vi "Load Single Level.vi"(8 "error in (no error)":errorcluster, 10 "Tag":string, 11 "TreeDirectory in":refnum<class "TreeDirectoryExt.lvclass">) -> (0 "error out":errorcluster, 3 "Tree (dup)":refnum<class "TreeDirectoryExt.lvclass">)   [LabVIEW 2026, in "TreeDirectoryExt.lvclass"]
uses:
  TreeDirectoryExt.lvclass
  C:/Program Files/National Instruments/LabVIEW 2026/vi.lib/QSI/QControls/QControl Classes/TreeControl/TreeControl.lvclass
  <vilib>/QSI/QControls/QControl Classes/TreeControl/Add Item Info Cluster.ctl
  TreeDirectoryExt.lvclass/TreeDirectoryExt.ctl
  <vilib>/QSI/QControls/QControl Classes/TreeControl/Tree Action Enum.ctl
  <vilib>/QSI/QControls/QControl Classes/TreeControl/TreeControl.lvclass
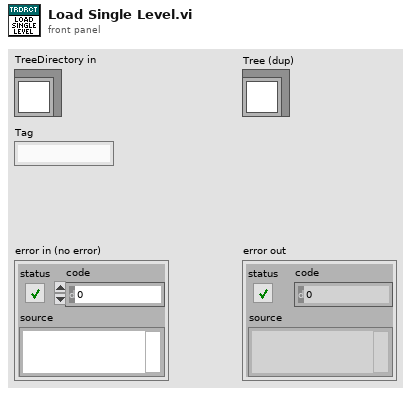
[diagram p1: front panel]
types:
  T1 = typedef "TreeControl.lvclass/Add Item Info Cluster.ctl" = cluster{"Parent Tag (\"\")":string, "Child Position (-1=End)":i32, "Left Cell String (\"\" = Same as Child Tag)":string, "Child Text[]":string[], "Child Tag":string, "Child Only? (F)":bool}
  T2 = typedef "TreeControl.lvclass/Tree Action Enum.ctl" = enum16{"Open All", "Close All", "Open Item", "Close Item"}
  T3 = typedef "imagedata.ctl" = cluster{"image type":i32, "image depth":i32, "image":u8[], "mask":u8[], "colors":u32[], "Rectangle":cluster{"left":i16, "top":i16, "right":i16, "bottom":i16}}
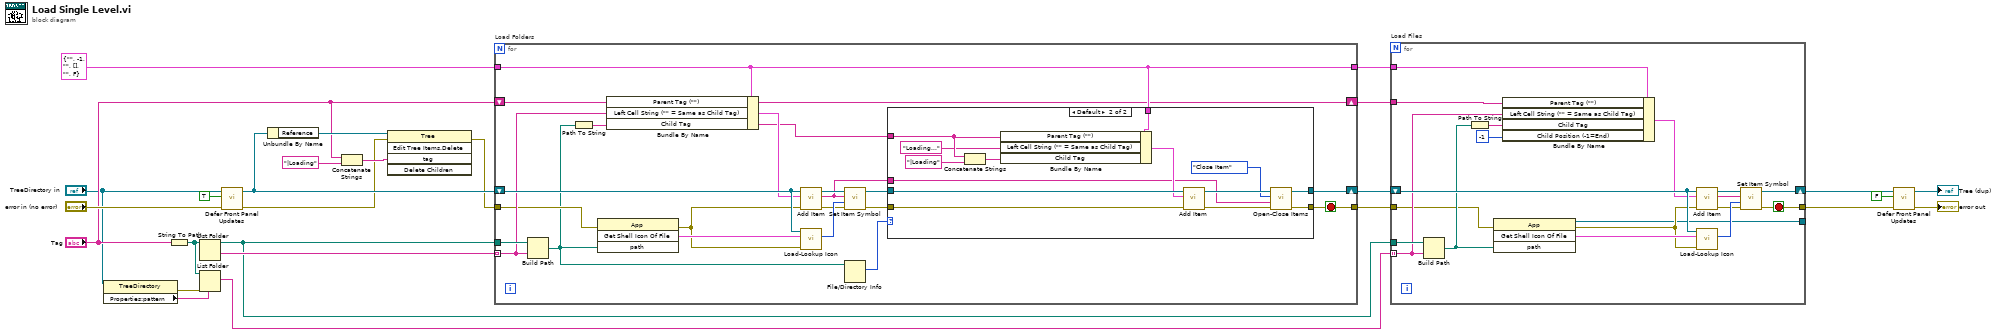
[diagram p0: block diagram]
diagram:
  n1 = property class="TreeDirectory"(reference="TreeDirectory in") -> (error out=w1:errorcluster, "Properties:pattern"=w2:string)  [unwired: 1 in, 1 out]
  n2 = String To Path(string="Tag") -> (path=w5:path)
  n3 = List Folder(path=w5) -> (path out=w21:path, folder names=w26:string[])  [unwired: 3 in, 2 out]
  n4 = List Folder(path=w5, pattern=w2, error in=w1) -> (filenames=w4:string[])  [unwired: 1 in, 3 out]
  n5 = call <vilib>:"Defer Front Panel Updates.vi"("error in (no error)"="error in (no error)", "Defer Panel Updates (F)"=TRUE, "Tree in"="TreeDirectory in") -> ("error out"=w13:errorcluster, "Tree (dup)"=w17:refnum<class "TreeDirectoryExt.lvclass">)  [unwired: 7 in]
  n6 = Unbundle By Name(w17) -> ("Reference"=w16:refnum<vi>)
  n7 = Concatenate Strings("Tag", "|Loading" ("string")) -> (w14:string)
  n8 = invoke class="Tree" method="Edit Tree Items.Delete"(reference=w16, error in=w13, "tag"=w14) -> (error out=w12:errorcluster)  [unwired: 2 in, 4 out]
  n9 = for "Load Folders" {
    tunnel: w26 -> [w42] mode=indexing
    shift-right: [w34] -> w25
    shift-left: w17 -> [w44]
    tunnel: w21 -> [w46]
    tunnel: T1 {"Parent Tag (\"\")"="", "Child Position (-1=End)"=-1, "Left Cell String (\"\" = Same as Child Tag)"="", "Child Text[]"=[], "Child Tag"="", "Child Only? (F)"=FALSE} ("ItemInfo") -> [w36]
    tunnel: [w36] -> w23
    tunnel: [w33] -> w7
    tunnel: w12 -> [w32]
    shift-right: [w29] -> w22
    shift-left: "Tag" -> [w29]
    stop <- w33 stop-if-true
    n10 = Build Path(base path=w46, name or relative path=w42) -> (appended path=w28:path)
    n11 = Path To String(path=w28) -> (string=w40:string)
    n12 = invoke class="App" method="Get Shell Icon Of File"(error in=w32, "path"=w28) -> (error out=w30:errorcluster, "GetShellIconOfFile"=w31:T3)  [unwired: 2 in, 2 out]
    n13 = Bundle By Name(cluster=w36, "Parent Tag (\"\")"=w29, "Left Cell String (\"\" = Same as Child Tag)"=w42, "Child Tag"=w40) -> (w41:T1)
    n14 = call-dynamic "Add Item.vi"("error in (no error)"=w30, "ItemInfo"=w41, "Tree in"=w44) -> ("error out"=w37:errorcluster, "Add Item Tag"=w35:string, "Tree (dup)"=w43:refnum<class "TreeDirectoryExt.lvclass">)  [unwired: 6 in]
    n15 = call "Load-Lookup Icon.vi"("error in (no error)"=w30, "Shell Icon"=w31, "TreeDirectory in"=w44) -> ("Icon Index"=w45:i32)  [unwired: 6 in, 2 out]
    n16 = call <vilib>:"Set Item Symbol.vi"("error in (no error)"=w37, "Symbol Index"=w45, "Tag"=w35, "Tree in"=w43) -> ("error out"=w38:errorcluster, "Tree (dup)"=w39:refnum<class "TreeDirectoryExt.lvclass">)  [unwired: 6 in]
    n17 = File/Directory Info(path=w28) -> (size=w27:i64)  [unwired: 1 in, 6 out]
    n18 = case shown="Default" w27 {
      tunnel: w40 -> [_ w62]
      tunnel: w39 -> [w48 w58]
      tunnel: w38 -> [w47 w56]
      tunnel: w36 -> [_ w55]
      tunnel: w35 -> [_ w52]
      tunnel: [w48 w50] -> w34
      tunnel: [w47 w49] -> w33
      frame 0 {
      }
      frame Default {
        n19 = Concatenate Strings(w62, "|Loading" ("string")) -> (w60:string)
        n20 = Bundle By Name(cluster=w55, "Parent Tag (\"\")"=w62, "Left Cell String (\"\" = Same as Child Tag)"="Loading..." ("string"), "Child Tag"=w60) -> (w57:T1)
        n21 = call-dynamic "Add Item.vi"("error in (no error)"=w56, "ItemInfo"=w57, "Tree in"=w58) -> ("error out"=w51:errorcluster, "Tree (dup)"=w54:refnum<class "TreeDirectoryExt.lvclass">)  [unwired: 6 in, 1 out]
        n22 = call-dynamic "Open-Close Items.vi"("error in (no error)"=w51, "Tag (\"\")"=w52, "Action (Close All)"=Tree_Action_Enum."Close Item", "Tree in"=w54) -> ("error out"=w49:errorcluster, "Tree (dup)"=w50:refnum<class "TreeDirectoryExt.lvclass">)  [unwired: 6 in]
      }
    }
  }
  n23 = for "Load Files" {
    tunnel: w4 -> [w75] mode=indexing
    shift-right: [w68] -> w18
    shift-left: w25 -> [w78]
    tunnel: w21 -> [w81]
    tunnel: w23 -> [w72]
    tunnel: w22 -> [w69]
    tunnel: w7 -> [w67]
    tunnel: [w65] -> w8
    tunnel: [w64] -> _
    stop <- w65 stop-if-true
    n24 = Build Path(base path=w81, name or relative path=w75) -> (appended path=w74:path)
    n25 = Path To String(path=w74) -> (string=w71:string)
    n26 = invoke class="App" method="Get Shell Icon Of File"(error in=w67, "path"=w74) -> (reference out=w64:refnum<vi>, error out=w66:errorcluster, "GetShellIconOfFile"=w80:T3)  [unwired: 2 in, 1 out]
    n27 = Bundle By Name(cluster=w72, "Parent Tag (\"\")"=w69, "Left Cell String (\"\" = Same as Child Tag)"=w75, "Child Tag"=w71, "Child Position (-1=End)"=-1) -> (w73:T1)
    n28 = call-dynamic "Add Item.vi"("error in (no error)"=w66, "ItemInfo"=w73, "Tree in"=w78) -> ("error out"=w70:errorcluster, "Add Item Tag"=w76:string, "Tree (dup)"=w77:refnum<class "TreeDirectoryExt.lvclass">)  [unwired: 6 in]
    n29 = call "Load-Lookup Icon.vi"("error in (no error)"=w66, "Shell Icon"=w80, "TreeDirectory in"=w78) -> ("Icon Index"=w79:i32)  [unwired: 6 in, 2 out]
    n30 = call <vilib>:"Set Item Symbol.vi"("error in (no error)"=w70, "Symbol Index"=w79, "Tag"=w76, "Tree in"=w77) -> ("error out"=w65:errorcluster, "Tree (dup)"=w68:refnum<class "TreeDirectoryExt.lvclass">)  [unwired: 6 in]
  }
  n31 = call <vilib>:"Defer Front Panel Updates.vi"("error in (no error)"=w8, "Defer Panel Updates (F)"=FALSE, "Tree in"=w18) -> ("error out"=→"error out":errorcluster, "Tree (dup)"=→"Tree (dup)":refnum<class "TreeDirectoryExt.lvclass">)  [unwired: 7 in]
